vi "PackagePython.vi"() -> ()   [LabVIEW 2018]
panel:
  out "得到 Python 脚本的路径":path
  out "Application Directory":path caption="当前应用程序目录"
  in  "输出 hi 的个数":i32=20
  out "当前 VI 路径":path
  out "得到 Python 脚本的路径":path
  out "返回值":string
  out "应用程序:名称":string
  out "应用程序:目录路径":path
  out "应用程序:类别":T1(ring)
  # "Debug 信息"
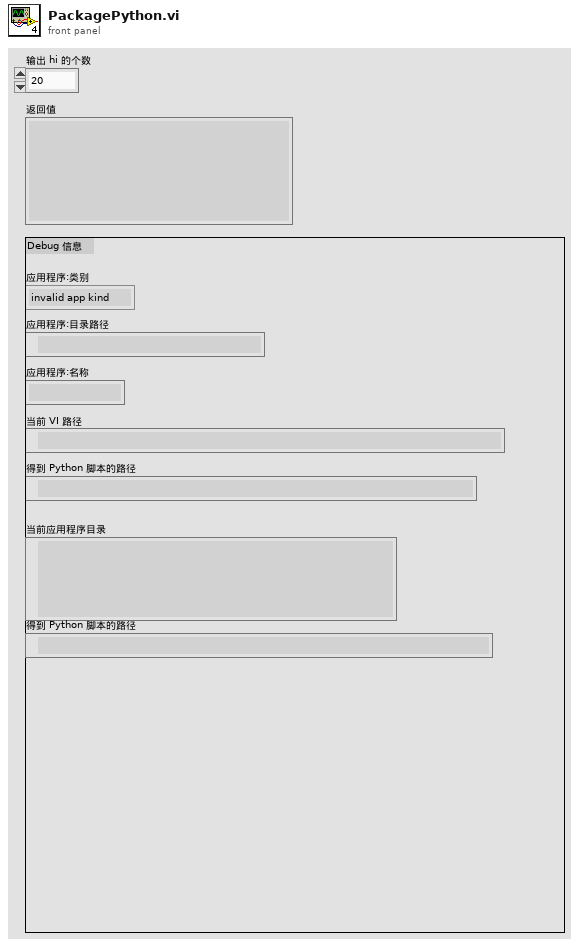
[diagram p1: front panel]
types:
  T1 = enum32{"invalid app kind", "Development System", "Run Time System", "Student Edition", "Embedded LabVIEW", "Evaluation", "Custom"}
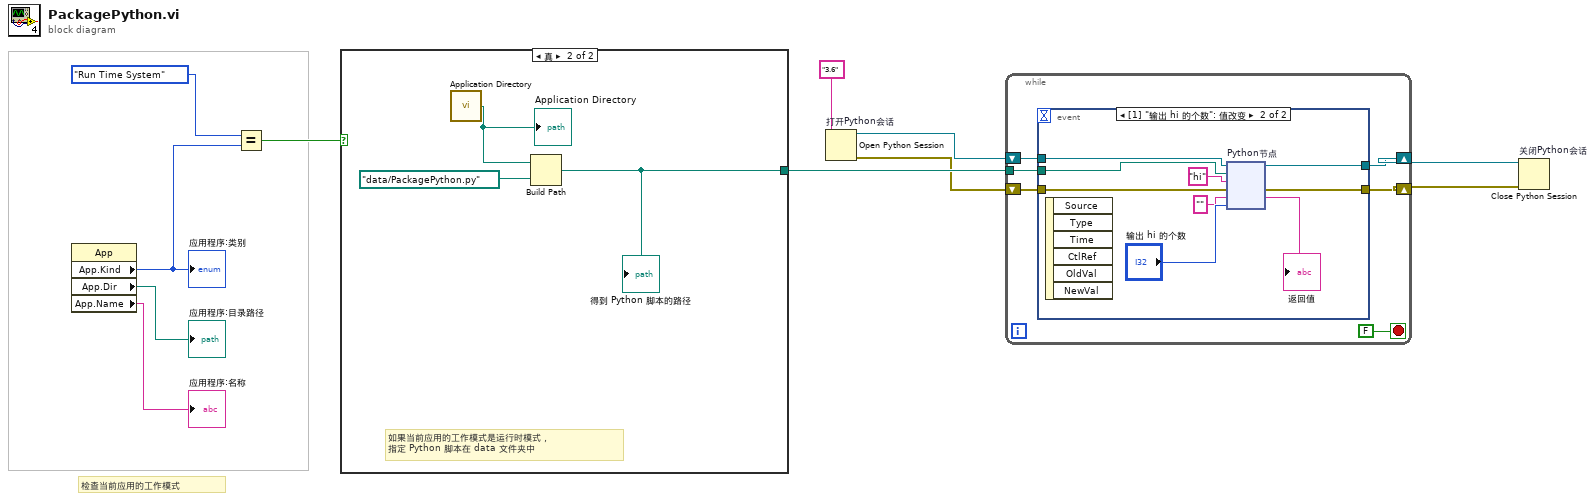
[diagram p0: block diagram]
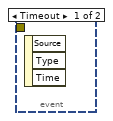
[diagram p2: hidden frame]
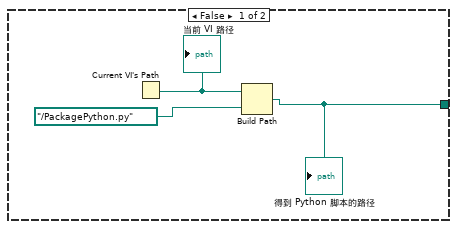
[diagram p3: hidden frame]
diagram:
  # "检查当前应用的工作模式"
  n1 = property class="App"() -> ("App.Kind"=w8:T1, "App.Dir"=→"应用程序:目录路径":path, "App.Name"=→"应用程序:名称":string)  [unwired: 2 in, 2 out]
  "应用程序:类别" <- w8
  n2 = Equal?(x=T1."Run Time System" ("应用程序:类别"), y=w8) -> (x = y?=w7:bool)
  n3 = case shown="真" w7 {
    tunnel: [w12 w16] -> w4
    frame False {
      n4 = Current VI's Path() -> (path=w14:path)
      "当前 VI 路径" <- w14
      n5 = Build Path(base path=w14, name or relative path=path "../PackagePython.py") -> (appended path=w12:path)
      "得到 Python 脚本的路径" <- w12
    }
    frame True {
      # "如果当前应用的工作模式是运行时模式，\n指定 Python 脚本在 data 文件夹中"
      n6 = call <vilib>:"Application Directory.vi"() -> ("Application Directory"=w15:path)
      "Application Directory" <- w15
      n7 = Build Path(base path=w15, name or relative path=path "data/PackagePython.py") -> (appended path=w16:path)
      "得到 Python 脚本的路径" <- w16
    }
  }
  n8 = Open Python Session "打开Python会话"(python version="3.6") -> (session out=w5:refnum<k35>, error out=w3:errorcluster)  [unwired: 2 in]
  n9 = while {
    tunnel: w4 -> [w22]
    shift-right: [w20] -> w2
    shift-left: w5 -> [w23]
    shift-right: [w19] -> w1
    shift-left: w3 -> [w21]
    stop <- FALSE stop-if-true
    n10 = event shown="[1] \"输出 hi 的个数\": 值改变" {
      selector: _ -> [_ _]
      dyn-events: _ -> [_ _]
      timeout: _ -> [_ _]
      tunnel: w23 -> [_ w30]
      tunnel: w22 -> [_ w29]
      tunnel: w21 -> [_ w27]
      tunnel: [_ w25] -> w20
      tunnel: [_ w24] -> w19
      event Timeout {
        n11 = event-data() -> ()  [unwired: 1 in, 3 out]
      }
      event "输出 hi 的个数": Value Change {
        n12 = event-data() -> ()  [unwired: 1 in, 6 out]
        n13 = node "Python节点"(w30, w29, "hi" ("函数名称"), w27, "", "输出 hi 的个数") -> (w25:refnum<k35>, w24:errorcluster, →"返回值":string)  [unwired: 1 in, 2 out]
      }
    }
  }
  n14 = Close Python Session "关闭Python会话"(session in=w2, error in=w1) -> ()  [unwired: 1 out]
